vi "Initialize.vi"(8 "error in (no error)":errorcluster, 9 "Reset (True)":bool=TRUE, 10 "ID Query (True)":bool=TRUE, 11 "VISA resource name":refnum<visa-resource-name>) -> (0 "error out":errorcluster, 3 "VISA resource name out":refnum<visa-resource-name>)   [LabVIEW 2020, in "Library Instrument & Equipement.lvlib" / "Library Power_Supply.lvlib" / "RIGOL DP800 Series.lvlib"]
doc: "Establishes communication with the instrument and optionally performs an instrument identification query and/or an instrument reset. It also places the instrument in a default state needed for other instrument driver operations. Therefore, call this VI before calling other instrument driver VIs for this instrument. Generally, you need to call the Initialize VI only once at the beginning of an application."
uses:
  RIGOL DP800 Series.lvlib
  4bacb4e6-58c4-4720-a790-12b92a79574c.vi
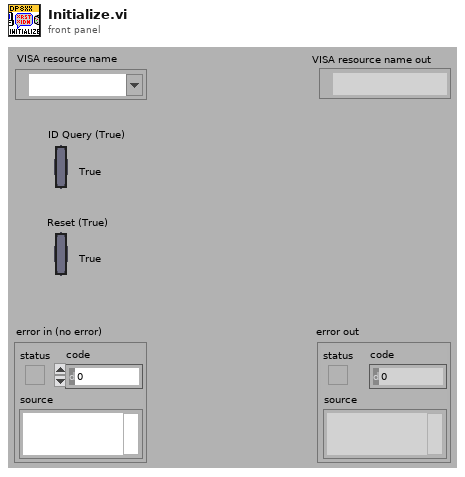
[diagram p1: front panel]
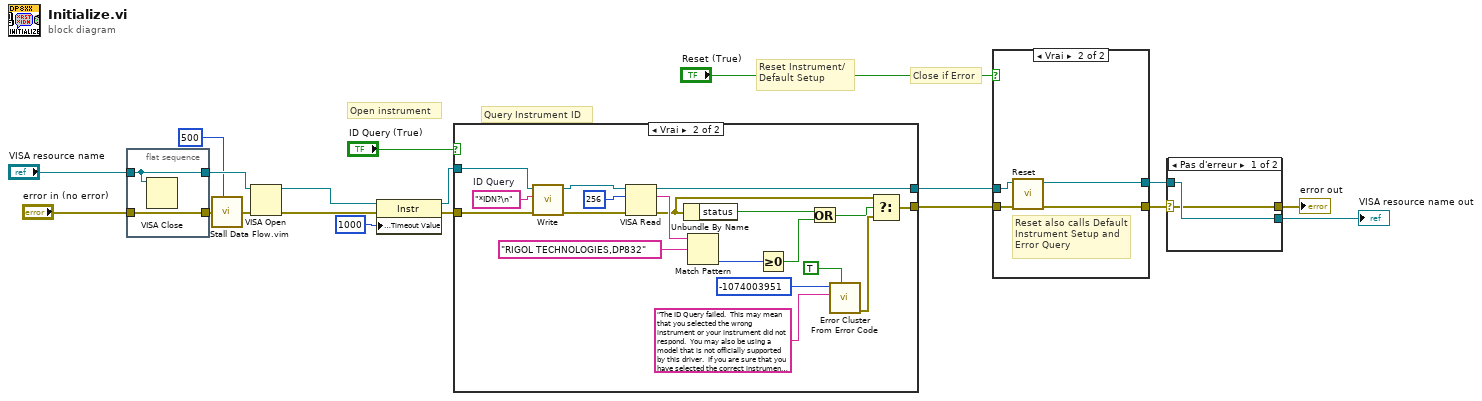
[diagram p0: block diagram]
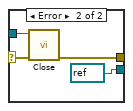
[diagram p2: hidden frame]
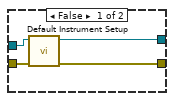
[diagram p3: hidden frame]
diagram:
  # "Close if Error"
  # "Query Instrument ID"
  # "Reset Instrument/\nDefault Setup"
  # "Open instrument"
  n1 = flat-sequence {
    tunnel: [w21] -> w6
    tunnel: "error in (no error)" -> [w21]
    tunnel: "VISA resource name" -> [w20]
    tunnel: [w20] -> w5
    frame #0 {
      n2 = VISA Close(VISA resource name=w20) -> ()  [unwired: 1 in, 1 out]
    }
  }
  n3 = call "Stall Data Flow.vim"("value in"=w6, "milliseconds to wait"=u32 500) -> ("value out"=w2:errorcluster)  [unwired: 1 out]
  n4 = VISA Open(error in (no error)=w2, VISA resource name=w5) -> (VISA resource name=w3:refnum<visa-resource-name>, error out=w4:errorcluster)  [unwired: 1 in, 2 out]
  n5 = property class="Instr"(reference=w3, error in=w4, "General Settings:Timeout Value"=u32 1000) -> (reference out=w10:refnum<visa-resource-name>, error out=w9:errorcluster)
  n6 = case shown="Vrai" "ID Query (True)" {
    tunnel: [w22 w42] -> w18
    tunnel: [w23 w41] -> w19
    tunnel: w10 -> [w23 w27]
    tunnel: w9 -> [w22 w28]
    frame False {
    }
    frame True {
      w26 = "*IDN?\n"  # ID Query
      n7 = call "Write.vi"("error in (no error)"=w28, "Write Buffer (\"\")"=w26, "VISA resource name"=w27) -> ("error out"=w29:errorcluster, "VISA resource name out"=w24:refnum<visa-resource-name>)  [unwired: 7 in]
      n8 = VISA Read(VISA resource name=w24, byte count=u32 256, error in (no error)=w29) -> (VISA resource name out=w41:refnum<visa-resource-name>, read buffer=w40:string, error out=w33:errorcluster)  [unwired: 1 out]
      n9 = Unbundle By Name(w33) -> ("status"=w32:bool)
      n10 = Match Pattern(string=w40, regular expression="RIGOL TECHNOLOGIES,DP832") -> (offset past match=w34:i32)  [unwired: 4 out]
      n11 = Greater Or Equal To 0?(x=w34) -> (x >= 0?=w31:bool)
      n12 = Or(x=w32, y=w31) -> (x .or. y?=w30:bool)
      n13 = call <vilib>:"Error Cluster From Error Code.vi"("show call chain? (False)"=TRUE, "error message (\"\")"="The ID Query failed.  This may mean that you selected the wrong instrument or your instrument did not respond.  You may also be using a model that is not officially supported by this driver.  If you are sure that you have selected the correct instrument and it is responding, try disabling the ID Query." ("Source (VI Name)"), "error code (0)"=-1074003951 ("Code")) -> ("error out"=w38:errorcluster)  [unwired: 1 in, 5 out]
      n14 = Select(t=w33, s=w30, f=w38) -> (s? t:f=w42:errorcluster)
    }
  }
  n15 = case shown="Vrai" "Reset (True)" {
    tunnel: w18 -> [w45 w47]
    tunnel: [w43 w50] -> w11
    tunnel: w19 -> [w46 w48]
    tunnel: [w44 w49] -> w12
    frame False {
      n16 = call "Default Instrument Setup.vi"("error in (no error)"=w45, "VISA resource name"=w46) -> ("error out"=w43:errorcluster, "VISA resource name out"=w44:refnum<visa-resource-name>)  [unwired: 8 out]
    }
    frame True {
      # "Reset also calls Default Instrument Setup and Error Query"
      n17 = call "Reset.vi"("error in (no error)"=w47, "VISA resource name"=w48) -> ("error out"=w50:errorcluster, "VISA resource name out"=w49:refnum<visa-resource-name>)  [unwired: 8 out]
    }
  }
  n18 = case shown="Pas d'erreur" w11 {
    selector: w11 -> [w51 w54]
    tunnel: w12 -> [w52 w55]
    tunnel: [w52 refnum<visa-resource-name> refnum ("VISA resource name out")] -> w14
    tunnel: [w51 w56] -> w13
    frame No Error {
    }
    frame Error {
      n19 = call "Close.vi"("error in (no error)"=w54, "VISA resource name"=w55) -> ("error out"=w56:errorcluster)  [unwired: 9 out]
    }
  }
  "VISA resource name out" <- w14
  "error out" <- w13
